vi "Time.vi"(8 "error in (no error)":errorcluster, 10 "Control In":T1={"I-O.lvclass"=refnum, "Motion.lvclass"=refnum, "Dispenser.lvclass"=refnum}, 11 "CAD Dispense in":refnum<class "CAD Dispense.lvclass">) -> (0 "error out":errorcluster, 1 "Timing Data":i32[](array[numeric]), 2 "Control Out":T1, 3 "CAD Dispense out":refnum<class "CAD Dispense.lvclass">)   [LabVIEW 2016, in "CAD Dispense.lvclass"]
uses:
  CAD Dispense.lvclass
  Controller/Controllers.ctl
  Controller/I-O/I-O.lvclass
  Controller/Motion/A3200/A3200.lvclass
  Controller/Dispenser/Dispenser.lvclass
  Controller/Motion/Motion.lvclass
  CAD Dispense.lvclass/CAD Dispense.ctl
  Controller/Controller.lvclass
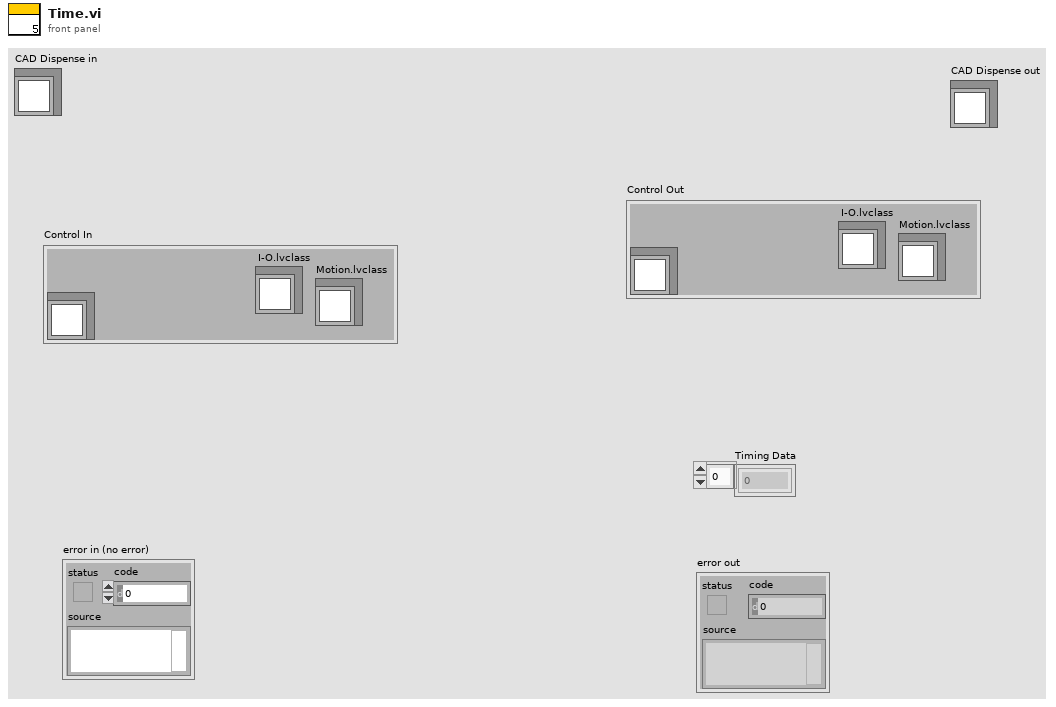
[diagram p1: front panel]
types:
  T1 = typedef "Controller.lvclass/Controllers.ctl" = cluster{"I-O.lvclass":refnum<class "I-O.lvclass">, "Motion.lvclass":refnum<class "Motion.lvclass">, "Dispenser.lvclass":refnum<class "Dispenser.lvclass">}
  T2 = cluster{"Motion":dbl[][], "Center":dbl[], "Circle?":bool, "CW/CCW":dbl}[]
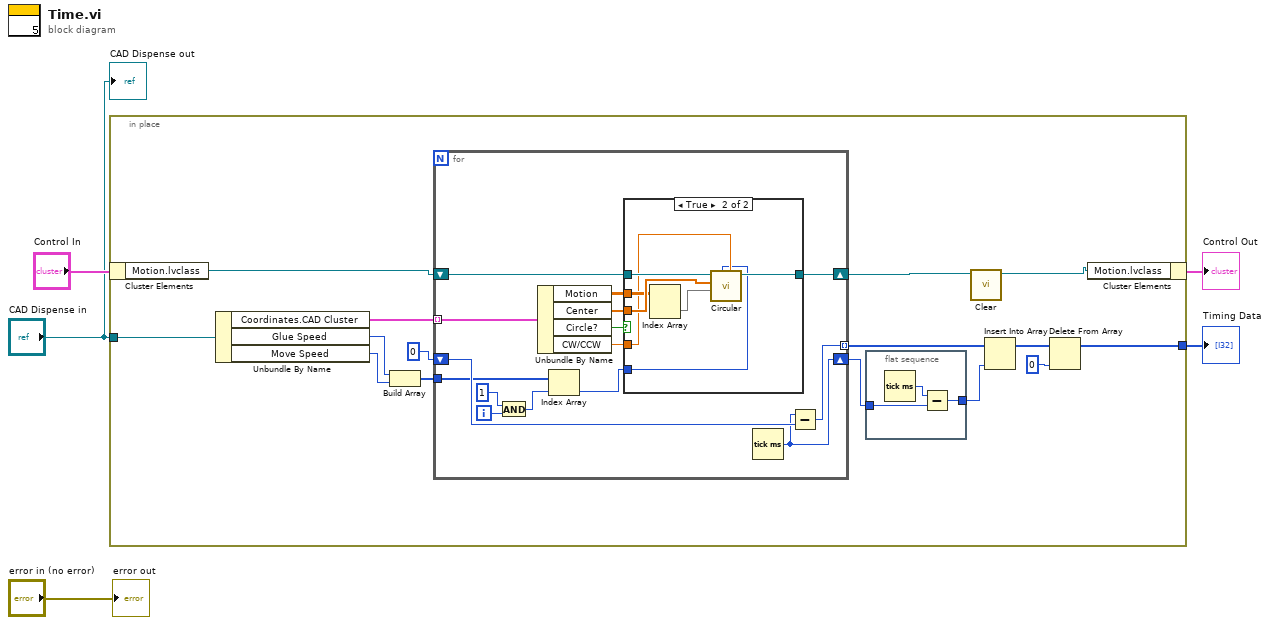
[diagram p0: block diagram]
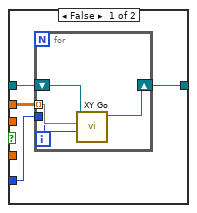
[diagram p2: hidden frame]
diagram:
  n1 = in-place {
    in-place-border: "CAD Dispense in" -> [w20]
    in-place-border: [w9] -> w1
    n2 = in-place-cluster #1("Control In") -> ("Motion.lvclass"=w8:refnum<class "Motion.lvclass">)
    n3 = Unbundle By Name(w20) -> ("Coordinates.CAD Cluster"=w10:T2, "Glue Speed"=w12:i32, "Move Speed"=w11:i32)
    n4 = Build Array(w12, w11) -> (w13:i32[])
    n5 = for {
      shift-right: [w33] -> w14
      shift-left: u32 0 ("millisecond timer value") -> [w36]
      tunnel: [w35] -> w16 mode=indexing
      tunnel: w10 -> [w31] mode=indexing
      tunnel: w13 -> [w27]
      shift-right: [w24] -> w7
      shift-left: w8 -> [w25]
      i -> [w37]
      n6 = And(x=1, y=w37) -> (x .and. y?=w34:i32)
      n7 = Unbundle By Name(w31) -> ("Motion"=w30:dbl[][], "Center"=w29:dbl[], "Circle?"=w28:bool, "CW/CCW"=w26:dbl)
      n8 = Index Array(array=w27, index=w34) -> (element=w32:i32)
      n9 = case shown="True" w28 {
        tunnel: w32 -> [w42 w47]
        tunnel: [w39 w49] -> w24
        tunnel: w30 -> [w40 w52]
        tunnel: w29 -> [_ w53]
        tunnel: w26 -> [_ w48]
        tunnel: w25 -> [w41 w50]
        frame False {
          n10 = for {
            tunnel: w42 -> [w43]
            tunnel: w40 -> [w44] mode=indexing
            shift-right: [w45] -> w39
            shift-left: w41 -> [w46]
            n11 = call-dynamic "XY Go.vi"("Speed"=w43, "XY"=w44, "Motion in"=w46) -> ("Motion out"=w45:refnum<class "Motion.lvclass">)  [unwired: 7 in, 1 out]
          }
        }
        frame True {
          n12 = Index Array(array=w52) -> (element=w51:dbl[])  [unwired: 2 in]
          n13 = call-dynamic "Circular.vi"("Direction"=w48, "Speed"=w47, "XY End"=w51, "XY Center"=w53, "Motion in"=w50) -> ("Motion out"=w49:refnum<class "Motion.lvclass">)  [unwired: 5 in, 1 out]
        }
      }
      n14 = Tick Count (ms)() -> (millisecond timer value=w33:u32)
      n15 = Subtract(x=w33, y=w36) -> (x-y=w35:u32)
    }
    n16 = flat-sequence {
      tunnel: [w22] -> w17
      tunnel: w14 -> [w21]
      frame #0 {
        n17 = Tick Count (ms)() -> (millisecond timer value=w23:u32)
        n18 = Subtract(x=w23, y=w21) -> (x-y=w22:u32)
      }
    }
    n19 = call "Clear.vi"("Motion in"=w7) -> ("Motion out"=w6:refnum<class "Motion.lvclass">)  [unwired: 9 in, 1 out]
    n20 = Insert Into Array(array=w16, new element=w17) -> (w15:u32[])  [unwired: 1 in]
    n21 = Delete From Array(array=w15, index=0) -> (array with subset deleted=w9:u32[])  [unwired: 1 in, 1 out]
    n22 = in-place-cluster #1("Motion.lvclass"=w6) -> (→"Control Out":T1)
  }
  "Timing Data" <- w1
  "error out" <- "error in (no error)"
  "CAD Dispense out" <- "CAD Dispense in"
